vi "matriz_magica.vi"() -> ()   [LabVIEW 2021]
panel:
  out "x+y":i32
  out "temp":i32
  in  "nxm":i32
  out "Matrix":dbl[][](array[numeric])
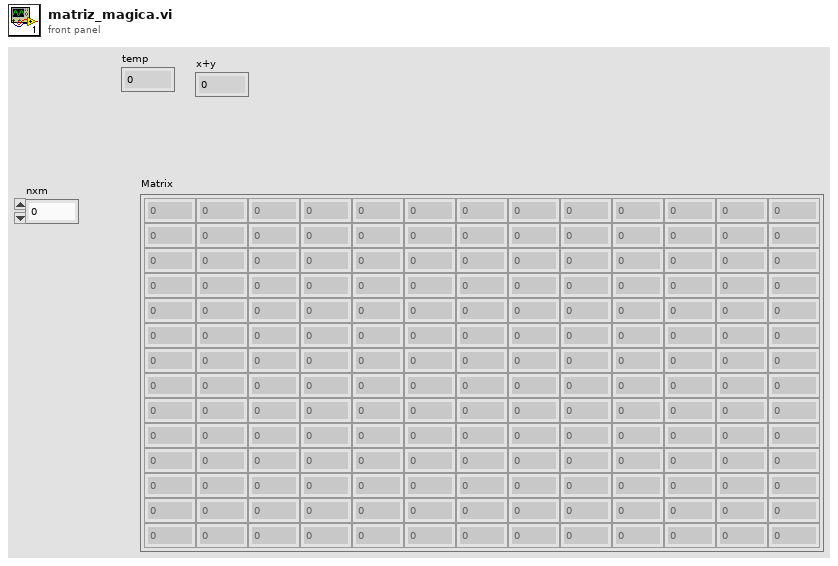
[diagram p1: front panel]
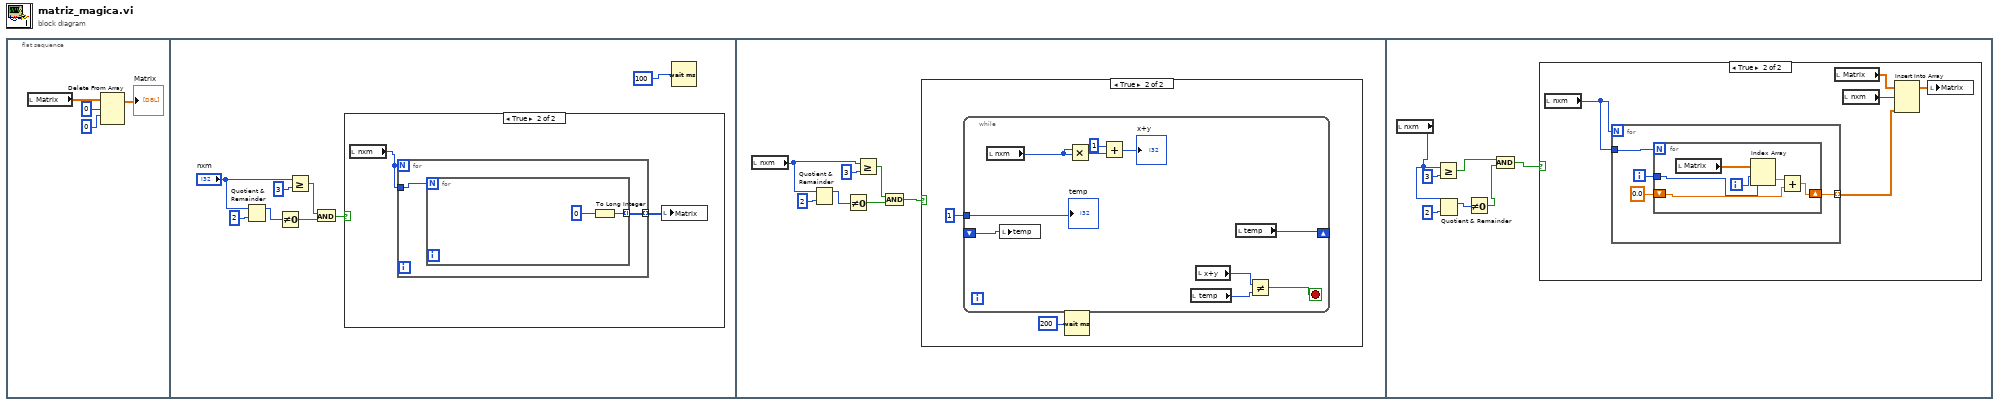
[diagram p0: block diagram]
diagram:
  n1 = flat-sequence {
    frame #0 {
      n2 = local read "Matrix"() -> (w2:dbl[][])
      n3 = Delete From Array(array=w2, length=0, index (row)=0) -> (array with subset deleted=→"Matrix":dbl[][])  [unwired: 1 in, 1 out]
    }
    frame #1 {
      n4 = Quotient & Remainder(x="nxm", y=2) -> (x-y*floor(x/y)=w6:i32)  [unwired: 1 out]
      n5 = Not Equal To 0?(x=w6) -> (x != 0?=w5:bool)
      n6 = Greater Or Equal?(x="nxm", y=3) -> (x >= y?=w8:bool)
      n7 = And(x=w8, y=w5) -> (x .and. y?=w7:bool)
      n8 = case shown="True" w7 {
        frame False {
        }
        frame True {
          n9 = local read "nxm"() -> (w13:i32)
          n10 = for {
            N: w13 -> [_]
            tunnel: [w16] -> w14 mode=indexing
            tunnel: w13 -> [w15]
            n11 = for {
              N: w15 -> [_]
              tunnel: [w18] -> w16 mode=indexing
              n12 = To Long Integer(number=0) -> (32bit integer=w18:i32)
            }
          }
          n13 = local write "Matrix"(w14) -> ()
        }
      }
      n14 = Wait (ms)(milliseconds to wait=u32 100) -> ()  [unwired: 1 out]
    }
    frame #2 {
      n15 = local read "nxm"() -> (w19:i32)
      n16 = Quotient & Remainder(x=w19, y=2) -> (x-y*floor(x/y)=w22:i32)  [unwired: 1 out]
      n17 = Not Equal To 0?(x=w22) -> (x != 0?=w21:bool)
      n18 = Greater Or Equal?(x=w19, y=3) -> (x >= y?=w23:bool)
      n19 = And(x=w23, y=w21) -> (x .and. y?=w20:bool)
      n20 = case shown="True" w20 {
        frame False {
        }
        frame True {
          n21 = while {
            tunnel: 1 -> [w30]
            shift-right: [w28] -> _
            shift-left: _ -> [w29]
            stop <- w31 stop-if-true
            n22 = local read "nxm"() -> (w37:i32)
            n23 = local write "temp"(w29) -> ()
            n24 = Multiply(x=w37, y=w37) -> (x*y=w36:i32)
            n25 = Add(x=1, y=w36) -> (x+y=→"x+y":i32)
            n26 = local read "temp"() -> (w32:i32)
            n27 = local read "x+y"() -> (w33:i32)
            n28 = local read "temp"() -> (w28:i32)
            n29 = Not Equal?(x=w33, y=w32) -> (x != y?=w31:bool)
            "temp" <- w30
          }
          n30 = Wait (ms)(milliseconds to wait=u32 200) -> ()  [unwired: 1 out]
        }
      }
    }
    frame #3 {
      n31 = local read "nxm"() -> (w38:i32)
      n32 = Greater Or Equal?(x=w38, y=3) -> (x >= y?=w42:bool)
      n33 = Quotient & Remainder(x=w38, y=2) -> (x-y*floor(x/y)=w43:i32)  [unwired: 1 out]
      n34 = Not Equal To 0?(x=w43) -> (x != 0?=w44:bool)
      n35 = And(x=w42, y=w44) -> (x .and. y?=w39:bool)
      n36 = case shown="True" w39 {
        frame False {
        }
        frame True {
          n37 = local read "nxm"() -> (w49:i32)
          n38 = for {
            N: w49 -> [_]
            tunnel: w49 -> [w53]
            tunnel: [w51] -> w46 mode=indexing
            i -> [w52]
            n39 = for {
              N: w53 -> [_]
              tunnel: w52 -> [w54]
              shift-right: [w57] -> w51
              shift-left: 0.0 -> [w58]
              i -> [w55]
              n40 = local read "Matrix"() -> (w59:dbl[][])
              n41 = Index Array(array=w59, index (row)=w55, index (col)=w54) -> (element=w56:dbl)
              n42 = Add(x=w56, y=w58) -> (x+y=w57:dbl)
            }
          }
          n43 = local read "Matrix"() -> (w48:dbl[][])
          n44 = local read "nxm"() -> (w45:i32)
          n45 = Insert Into Array(array=w48, index (row)=w45, new element=w46) -> (w47:dbl[][])  [unwired: 1 in]
          n46 = local write "Matrix"(w47) -> ()
        }
      }
    }
  }
